vi "Array2DLastNRows.vi"(1 "N":i32=950, 2 "Array in":dbl[][](array[numeric])) -> (0 "Array out":dbl[][](array[numeric]))   [LabVIEW 2014]
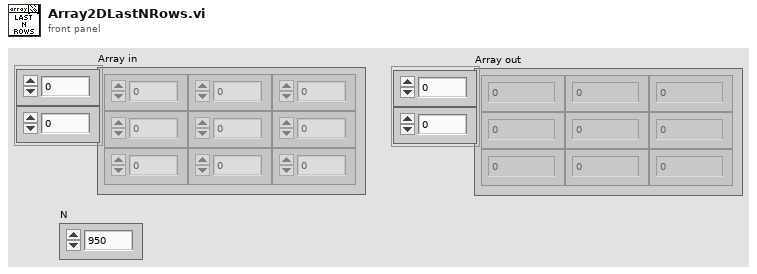
[diagram p1: front panel]
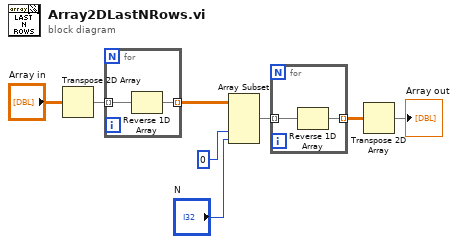
[diagram p0: block diagram]
diagram:
  n1 = Transpose 2D Array(2D array="Array in") -> (transposed array=w8:dbl[][])
  n2 = for {
    tunnel: w8 -> [w10] mode=indexing
    tunnel: [w9] -> w3 mode=indexing
    n3 = Reverse 1D Array(array=w10) -> (reversed array=w9:dbl[])
  }
  n4 = Array Subset(array=w3, index (col)=0 ("index"), length (col)="N") -> (w4:dbl[][])  [unwired: 2 in]
  n5 = for {
    tunnel: w4 -> [w12] mode=indexing
    tunnel: [w11] -> w6 mode=indexing
    n6 = Reverse 1D Array(array=w12) -> (reversed array=w11:dbl[])
  }
  n7 = Transpose 2D Array(2D array=w6) -> (transposed array=→"Array out":dbl[][])
